vi "Create Server Change Subscription.vi"(8 "error in (no error)":errorcluster, 11 "Client - Data":T1) -> (0 "error out":errorcluster, 3 "dup Client - Data":T1)   [LabVIEW 2024]
doc: "Creates a subscription to the server. When the server incurs changes, the client gets a notification."
uses:
  Controls/Client/Client - Data.ctl
  Shared/Message Queue/Client Message Queues.ctl
  Shared/Message Queue/Message Cluster.ctl
  <vilib>/lvdsc/NI_DSC.lvlib
  Shared/Message Queue.lvlib
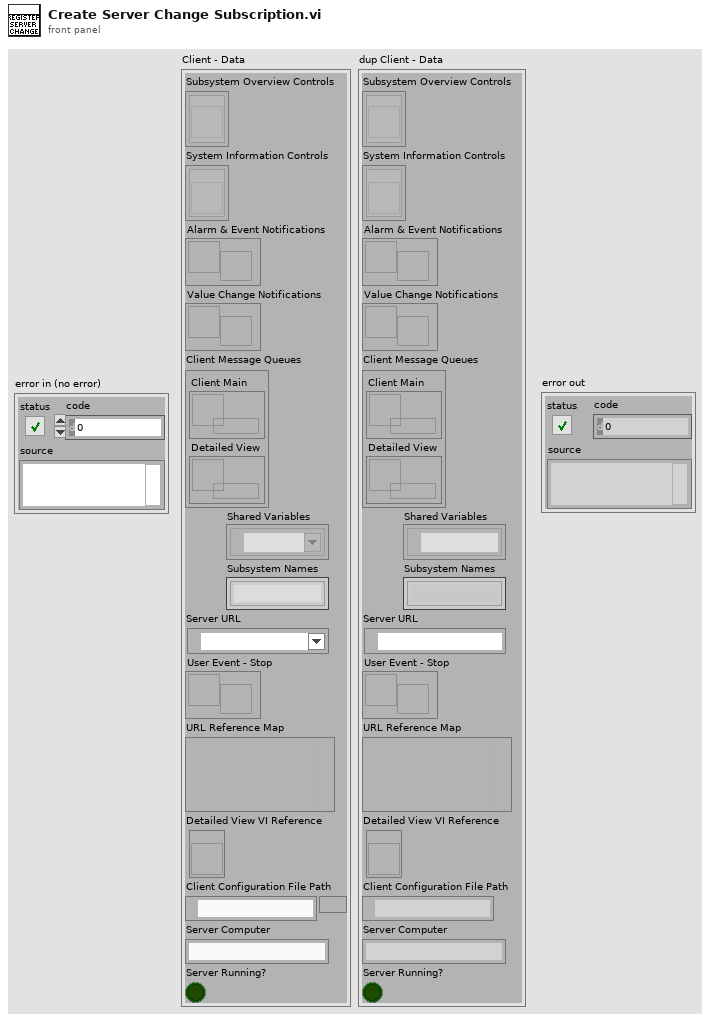
[diagram p1: front panel]
types:
  T1 = typedef "Client - Data.ctl" = cluster{"Subsystem Overview Controls":refnum<vi>[], "System Information Controls":refnum<vi>[], "Alarm & Event Notifications":refnum<user-event>, "Value Change Notifications":refnum<user-event>, "Client Message Queues":T2, "Shared Variables":refnum<k21>[], "Subsystem Names":string[], "Server URL":refnum<k21>, "User Event - Stop":refnum<user-event>, "URL Reference Map":variant, "Detailed View VI Reference":refnum<vi>, "Client Configuration File Path":path, "Server Computer":string, "Server Running?":bool}
  T2 = typedef "Message Queue.lvlib/Client Message Queues.ctl" = cluster{"Client Main":refnum<queue>, "Detailed View":refnum<queue>}
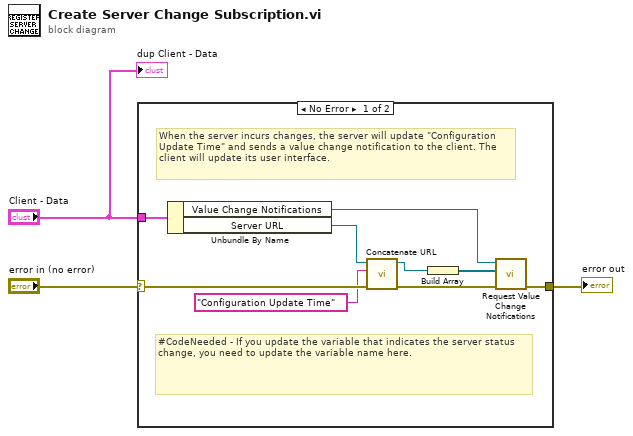
[diagram p0: block diagram]
diagram:
  n1 = case shown="No Error" "error in (no error)" {
    selector: "error in (no error)" -> [w8 w13]
    tunnel: [w9 w13] -> w2
    tunnel: "Client - Data" -> [w6 _]
    frame No Error {
      # "#CodeNeeded - If you update the variable that indicates the server status change, you need to update the variable name here."
      # "When the server incurs changes, the server will update \"Configuration Update Time\" and sends a value change notification to the client. The client will update its user interface."
      n2 = Unbundle By Name(w6) -> ("Value Change Notifications"=w4:refnum<user-event>, "Server URL"=w5:refnum<k21>)
      n3 = call "Concatenate URL.vi"("error in (no error)"=w8, "Child Name"="Configuration Update Time", "Parent URL"=w5) -> ("error out"=w12:errorcluster, "Child URL"=w11:refnum<k21>)  [unwired: 7 in]
      n4 = Build Array(w11) -> (w10:refnum<k21>[])
      n5 = call <vilib>:"Request Value Change Notifications.vi"("error in (no error)"=w12, "shared variables"=w10, "notification refnum"=w4) -> ("error out"=w9:errorcluster)  [unwired: 6 in, 2 out]
    }
    frame Error {
    }
  }
  "error out" <- w2
  "dup Client - Data" <- "Client - Data"
